vi "CSV text to String Array.vi"(7 "CSV_String":string) -> (8 "String_Array":string[][](array[string]))   [LabVIEW 2013]
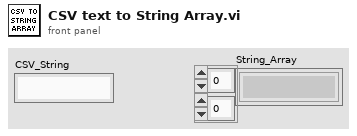
[diagram p1: front panel]
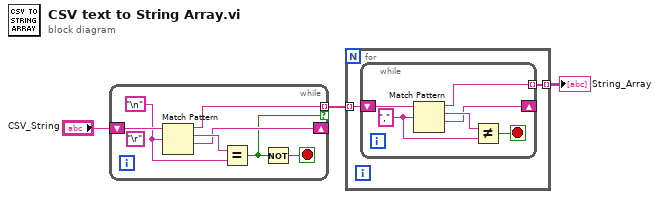
[diagram p0: block diagram]
diagram:
  n1 = while {
    shift-right: [w8] -> _
    shift-left: "CSV_String" -> [w10]
    tunnel: [w7] -> w2 mode=indexing if=w6
    stop <- w5 stop-if-true
    w4 = "\n"
    (unwired) "\r"
    n2 = Match Pattern(string=w10, regular expression=w4) -> (before substring=w7:string, match substring=w9:string, after substring=w8:string)  [unwired: 1 in, 1 out]
    n3 = Equal?(x=w9, y=w4) -> (x = y?=w6:bool)
    n4 = Not(x=w6) -> (.not. x?=w5:bool)
  }
  n5 = for {
    tunnel: w2 -> [w12] mode=indexing
    tunnel: [w11] -> w1 mode=indexing
    n6 = while {
      shift-right: [w16] -> _
      shift-left: w12 -> [w18]
      tunnel: [w15] -> w11 mode=indexing
      stop <- w13 stop-if-true
      w14 = ","
      n7 = Match Pattern(string=w18, regular expression=w14) -> (before substring=w15:string, match substring=w17:string, after substring=w16:string)  [unwired: 1 in, 1 out]
      n8 = Not Equal?(x=w17, y=w14) -> (x != y?=w13:bool)
    }
  }
  "String_Array" <- w1
